vi "lv_server.vi"() -> ()   [LabVIEW 2014]
uses:
  <vilib>/addons/zeromq/socket_type.ctl
  <vilib>/addons/zeromq/zmq_context.lvclass
  <vilib>/addons/zeromq/zmq_socket.lvclass
  <vilib>/addons/zeromq/zeromq.lvlib
panel:
  out "Message":string
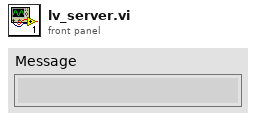
[diagram p1: front panel]
types:
  T1 = typedef "zeromq.lvlib/socket_type.ctl" = enum8{"ZMQ_PAIR", "ZMQ_PUB", "ZMQ_SUB", "ZMQ_REQ", "ZMQ_REP", "ZMQ_DEALER", "ZMQ_ROUTER", "ZMQ_PULL", "ZMQ_PUSH", "ZMQ_XPUB", "ZMQ_XSUB"}
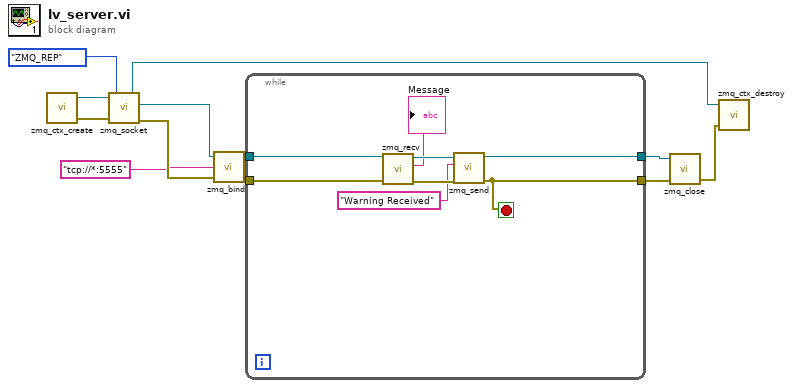
[diagram p0: block diagram]
diagram:
  n1 = call <vilib>:"zmq_ctx_create.vi"() -> ("error out"=w12:errorcluster, "context out"=w11:refnum<class "zmq_context.lvclass">)  [unwired: 4 in]
  n2 = call <vilib>:"zmq_socket.vi"("error in"=w12, "socket type"=socket_type."ZMQ_REP", "context in"=w11) -> ("error out"=w9:errorcluster, "socket out"=w3:refnum<class "zmq_socket.lvclass">, "context out"=w1:refnum<class "zmq_context.lvclass">)  [unwired: 2 in]
  n3 = call <vilib>:"zmq_bind.vi"("error in"=w9, "endpoint"="tcp://*:5555", "socket in"=w3) -> ("error out"=w6:errorcluster, "socket out"=w7:refnum<class "zmq_socket.lvclass">)  [unwired: 1 in]
  n4 = while {
    tunnel: w7 -> [w20]
    tunnel: [w16] -> w5
    tunnel: w6 -> [w19]
    tunnel: [w15] -> w4
    stop <- w15 stop-if-true
    n5 = call <vilib>:"zmq_recv.vi"("error in"=w19, "socket in"=w20) -> ("error out"=w18:errorcluster, "data"=→"Message":string, "socket out"=w14:refnum<class "zmq_socket.lvclass">)  [unwired: 3 in, 2 out]
    n6 = call <vilib>:"zmq_send.vi"("error in"=w18, "data"="Warning Received", "socket in"=w14) -> ("error out"=w15:errorcluster, "socket out"=w16:refnum<class "zmq_socket.lvclass">)  [unwired: 4 in]
  }
  n7 = call <vilib>:"zmq_close.vi"("error in"=w4, "socket"=w5) -> ("error out"=w2:errorcluster)  [unwired: 3 in]
  n8 = call <vilib>:"zmq_ctx_destroy.vi"("error in"=w2, "context in"=w1) -> ()  [unwired: 3 in, 1 out]
